vi "GetBoolValue.vi"(0 "nInputHandle":u64, 1 "strName":string, 2 "error in (no error)":errorcluster) -> (3 "nOutputHandle":u64, 4 "bValue":bool=TRUE, 5 "GX_STATUS":i32, 6 "error out":errorcluster)   [LabVIEW 2016, in "GxLVLib.lvlib"]
uses:
  GxLVLib.lvlib
  GxIAPI.dll
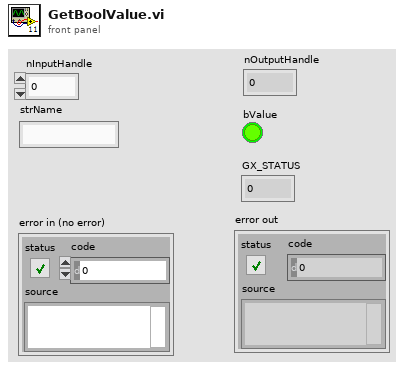
[diagram p1: front panel]
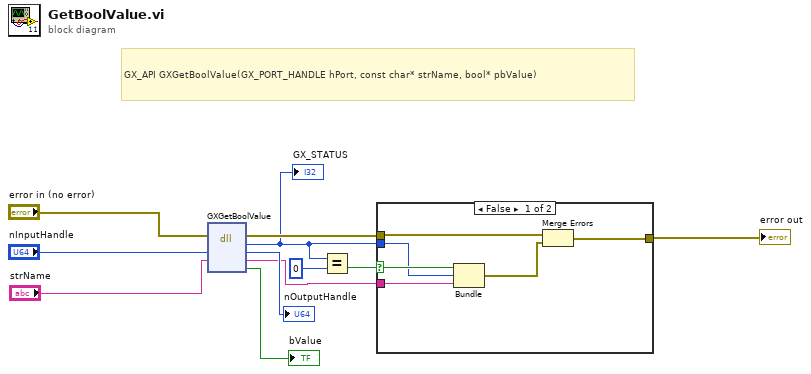
[diagram p0: block diagram]
diagram:
  # "GX_API GXGetBoolValue(GX_PORT_HANDLE hPort, const char* strName, bool* pbValue)"
  n1 = dll-call lib="GxIAPI.dll" fn="GXGetBoolValue"(error in="error in (no error)", "phDevice"="nInputHandle", "strName"="strName") -> (error out=w10:errorcluster, "GX_STATUS"=w5:i32, "phDevice"=→"nOutputHandle":i64, "strName"=w7:string, "bValue"=→"bValue":bool)  [unwired: 3 in, 1 out]
  "GX_STATUS" <- w5
  n2 = Equal?(x=w5, y=0) -> (x = y?=w8:bool)
  n3 = case shown="False" w8 {
    selector: w8 -> [w14 _]
    tunnel: w10 -> [w17 w18]
    tunnel: [w16 w18] -> w4
    tunnel: w5 -> [w13 _]
    tunnel: w7 -> [w12 _]
    frame False {
      n4 = Bundle(w14, "GX_STATUS"=w13, "strName"=w12) -> (w15:cluster{bool, "GX_STATUS":i32, "strName":string})  [unwired: 1 in]
      n5 = Merge Errors(w17, w15) -> (w16:errorcluster)
    }
    frame True {
    }
  }
  "error out" <- w4
